vi "FTW-ActorExtended-Publish.vi"(0 "FTW-ActorExtended In":refnum<class "FTW-ActorExtended.lvclass">, 5 "Publisher Name":string, 7 "Message Header":string, 9 "Message Body":string, 11 "error in":errorcluster) -> (4 "FTW-ActorExtended Out":refnum<class "FTW-ActorExtended.lvclass">, 15 "error out":errorcluster)   [LabVIEW 2013, in "FTW-ActorExtended.lvclass"]
uses:
  FTW-ActorExtended.lvclass
  FTW-ActorExtended.lvclass/FTW-ActorExtended.ctl
  Publisher/FTW-Publisher.lvclass
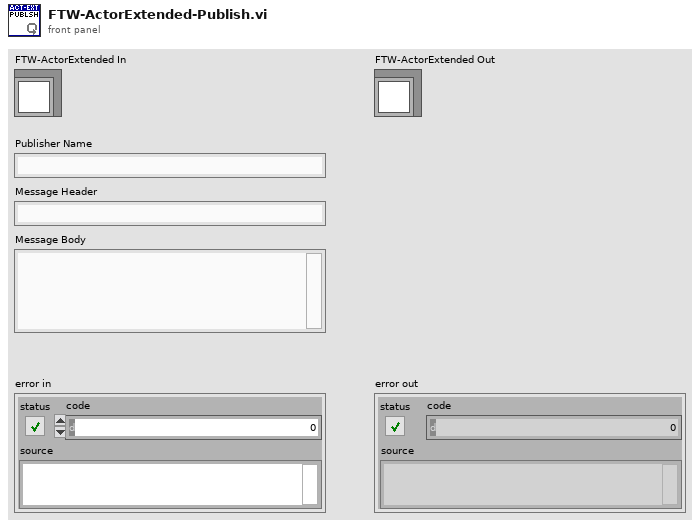
[diagram p1: front panel]
types:
  T1 = cluster{"Name":string, "URI":string, "FTW Publisher":refnum<class "FTW-Publisher.lvclass">}[]
  T2 = cluster{"Name":string, "URI":string, "FTW Publisher":refnum<class "FTW-Publisher.lvclass">}
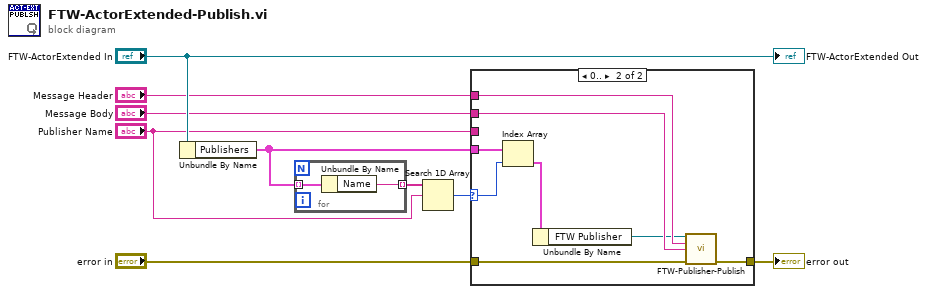
[diagram p0: block diagram]
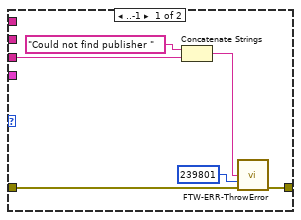
[diagram p2: hidden frame]
diagram:
  n1 = Unbundle By Name("FTW-ActorExtended In") -> ("Publishers"=w7:T1)
  n2 = for {
    tunnel: w7 -> [w11] mode=indexing
    tunnel: [w10] -> w1 mode=indexing
    n3 = Unbundle By Name(w11) -> ("Name"=w10:string)
  }
  n4 = Search 1D Array(1D array=w1, element="Publisher Name") -> (index of element=w8:i32)  [unwired: 1 in]
  n5 = case shown="0.." w8 {
    selector: w8 -> [_ w25]
    tunnel: w7 -> [_ w24]
    tunnel: [w16 w22] -> w6
    tunnel: "error in" -> [w17 w23]
    tunnel: "Publisher Name" -> [w12 _]
    tunnel: "Message Header" -> [_ w21]
    tunnel: "Message Body" -> [_ w20]
    frame ..-1 {
      n6 = Concatenate Strings("Could not find publisher " ("Error Message"), w12) -> (w13:string)
      n7 = call "FTW-ERR-ThrowError.vi"("Error Message"=w13, "Error Code"=239801, "error in"=w17) -> ("error out"=w16:errorcluster)  [unwired: 12 in]
    }
    frame 0.. {
      n8 = Index Array(array=w24, index=w25) -> (element=w19:T2)
      n9 = Unbundle By Name(w19) -> ("FTW Publisher"=w18:refnum<class "FTW-Publisher.lvclass">)
      n10 = call "FTW-Publisher-Publish.vi"("FTW-Publisher In"=w18, "Header"=w21, "Body"=w20, "error in"=w23) -> ("error out"=w22:errorcluster)  [unwired: 10 in, 1 out]
    }
  }
  "error out" <- w6
  "FTW-ActorExtended Out" <- "FTW-ActorExtended In"
